vi "Run.vi"(8 "error in (no error)":errorcluster, 9 "Penalty":dbl, 10 "Map":i32[][](array[numeric]), 11 "Runner in":refnum<class "Rain.lvclass">) -> (0 "error out":errorcluster, 1 "Direction":T2, 2 "Action":T3, 3 "Runner out":refnum<class "Rain.lvclass">, 4 "Replicated":refnum<class "Square.lvclass">)   [LabVIEW 2015, in "Rain.lvclass"]
uses:
  Rain.lvclass
  Type Defs/Action Enum.ctl
  Type Defs/Direction Enum.ctl
  Square/Square.lvclass
  Carl/Formics/Attack Options.ctl
  SubVIs/Read-Only Globals.vi
  Carl/Common/Common.lvlib
  Type Defs/SB Type Defs.lvlib
  Carl/Formics/Formics.lvclass
panel:
  in  "Attack":T1
  # "NOTICE - YOU MUST NOT REMOVE THIS NOTICE. PER THE FOLLOWING LICENSE, YOU MAY REPRODUCE THIS SOFTWARE PROVIDED YOU FOLLOW THE TERMS\nOF THE LICENSE.\n\n---BEGIN BSD LICENSE (http://opensource.org/licenses/BSD-2-Clause)---\nCopyright (c) 2015, Endigit, Inc. <robert@endigit.com>\nAll rights reserved.\n\nRedistribution and use in source and binary forms, with or without modification, are permitted provided that the following conditions are met:\n\n1. Redistributions of source code must retain the above copyright notice, this list of conditions and the following disclaimer.\n\n2. Redistributions in binary form must reproduce the above copyright notice, this list of conditions and the following disclaimer in the documentation and/or other \nmaterials provided with the distribution.\n\nTHIS SOFTWARE IS PROVIDED BY THE COPYRIGHT HOLDERS AND CONTRIBUTORS \"AS IS\" AND ANY EXPRESS OR IMPLIED WARRANTIES, INCLUDING, BUT NOT \nLIMITED TO, THE IMPLIED WARRANTIES OF MERCHANTABILITY AND FITNESS FOR A PARTICULAR PURPOSE ARE DISCLAIMED. IN NO EVENT SHALL THE COPYRIGHT \nHOLDER OR CONTRIBUTORS BE LIABLE FOR ANY DIRECT, INDIRECT, INCIDENTAL, SPECIAL, EXEMPLARY, OR CONSEQUENTIAL DAMAGES (INCLUDING, BUT NOT \nLIMITED TO, PROCUREMENT OF SUBSTITUTE GOODS OR SERVICES; LOSS OF USE, DATA, OR PROFITS; OR BUSINESS INTERRUPTION) HOWEVER CAUSED AND ON \nANY THEORY OF LIABILITY, WHETHER IN CONTRACT, STRICT LIABILITY, OR TORT (INCLUDING NEGLIGENCE OR OTHERWISE) ARISING IN ANY WAY OUT OF THE USE \nOF THIS SOFTWARE, EVEN IF ADVISED OF THE POSSIBILITY OF SUCH DAMAGE.\n---END BSD LICENSE---"
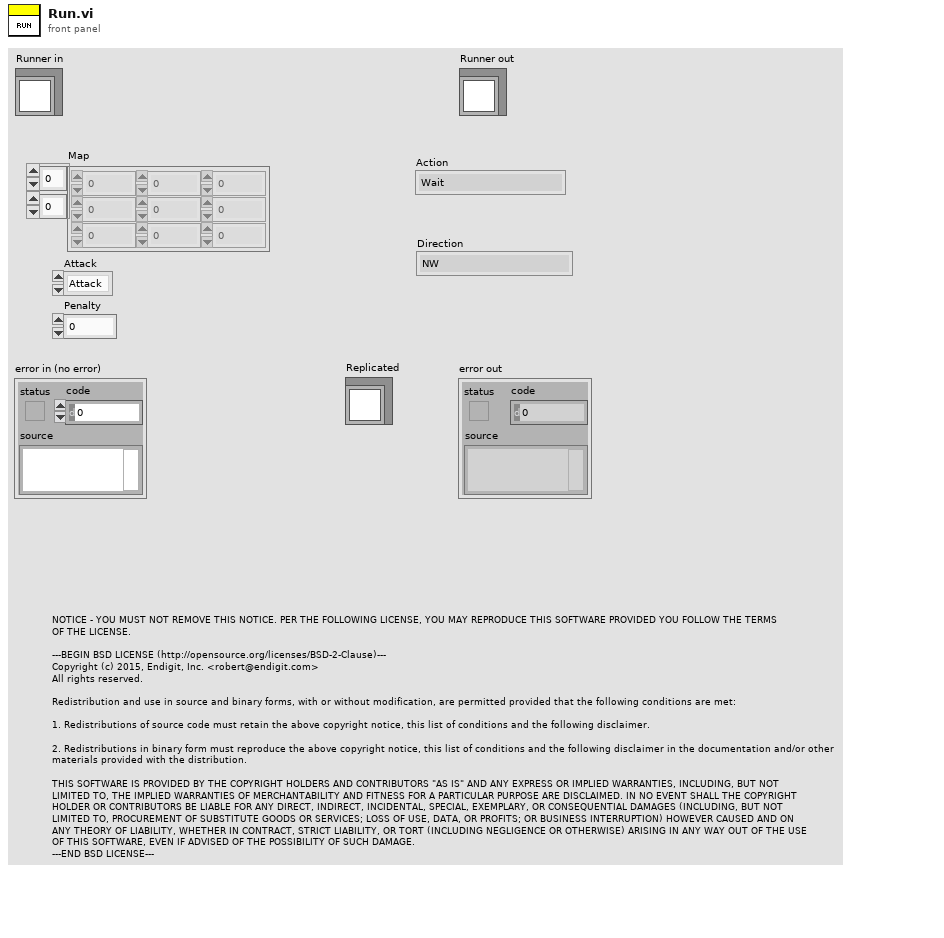
[diagram p1: front panel]
types:
  T1 = typedef "Formics.lvclass/Attack Options.ctl" = enum16{"Attack", "Run", "Distract"}
  T2 = typedef "SB Type Defs.lvlib/Direction Enum.ctl" = enum16{"NW", "N", "NE", "E", "SE", "S", "SW", "W"}
  T3 = typedef "SB Type Defs.lvlib/Action Enum.ctl" = enum16{"Wait", "Move", "Attack", "Replicate"}
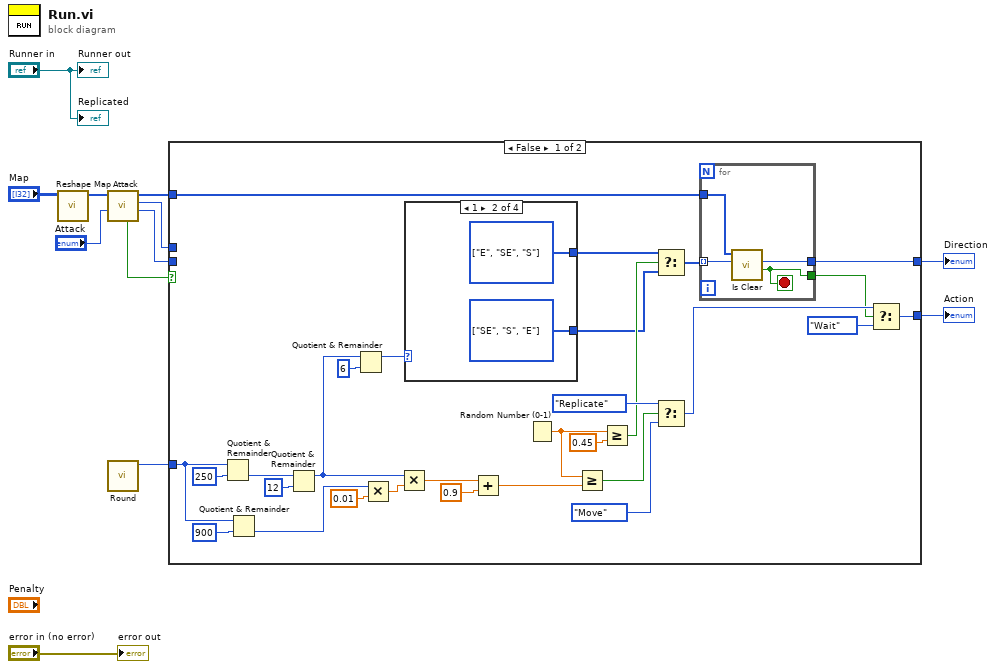
[diagram p0: block diagram]
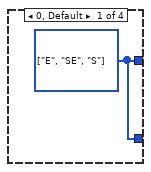
[diagram p2: hidden frame]
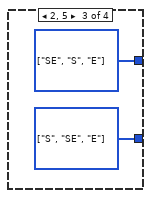
[diagram p3: hidden frame]
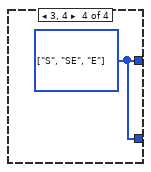
[diagram p4: hidden frame]
diagram:
  n1 = call "Reshape Map.vi"("Maze (0: Empty, -1: Enemy. >0: Teammate"="Map") -> ("Map"=w10:i32[])  [unwired: 9 in, 1 out]
  n2 = call "Attack.vi"("Attack?"="Attack", "Maze (0: Empty, -1: Enemy. >0: Teammate"=w10) -> ("Direction"=w8:i32, "Action"=w6:T3, "Maze (0: Empty, -1: Enemy. >0: Teammate 2"=w4:i32[], "Enemy Found?"=w9:bool)  [unwired: 4 in, 2 out]
  n3 = call "Round.vi"() -> ("Round"=w1:i32)  [unwired: 11 in]
  n4 = case shown="False" w9 {
    tunnel: w8 -> [_ w53]
    tunnel: [w34 w53] -> w7
    tunnel: w6 -> [_ w52]
    tunnel: [w38 w52] -> w5
    tunnel: w4 -> [w35 _]
    tunnel: w1 -> [w17 _]
    frame False {
      n5 = Quotient & Remainder(x=w17, y=250) -> (floor(x/y)=w25:i32)  [unwired: 1 out]
      n6 = Quotient & Remainder(x=w17, y=900) -> (floor(x/y)=w15:i32)  [unwired: 1 out]
      n7 = Quotient & Remainder(x=w25, y=12) -> (x-y*floor(x/y)=w19:i32)  [unwired: 1 out]
      n8 = Quotient & Remainder(x=w19, y=6) -> (x-y*floor(x/y)=w18:i32)  [unwired: 1 out]
      n9 = Multiply(x=w15, y=0.01) -> (x*y=w13:dbl)
      n10 = Multiply(x=w19, y=w13) -> (x*y=w24:dbl)
      n11 = case shown="1" w18 {
        tunnel: [w42 w44 w46 w47] -> w29
        tunnel: [w42 w43 w45 w47] -> w30
        frame 0, Default {
          w42 = T2[] [enum."E", enum."SE", enum."S"] items=["NW", "N", "NE", "E", "SE", "S", "SW", "W"]
        }
        frame 1 {
          w43 = T2[] [enum."SE", enum."S", enum."E"] items=["NW", "N", "NE", "E", "SE", "S", "SW", "W"]
          w44 = T2[] [enum."E", enum."SE", enum."S"] items=["NW", "N", "NE", "E", "SE", "S", "SW", "W"]
        }
        frame 2, 5 {
          w45 = T2[] [enum."S", enum."SE", enum."E"] items=["NW", "N", "NE", "E", "SE", "S", "SW", "W"]
          w46 = T2[] [enum."SE", enum."S", enum."E"] items=["NW", "N", "NE", "E", "SE", "S", "SW", "W"]
        }
        frame 3, 4 {
          w47 = T2[] [enum."S", enum."SE", enum."E"] items=["NW", "N", "NE", "E", "SE", "S", "SW", "W"]
        }
      }
      n12 = Add(x=w24, y=0.9) -> (x+y=w22:dbl)
      n13 = Random Number (0-1)() -> (number: 0 to 1=w27:dbl)
      n14 = Greater Or Equal?(x=w27, y=w22) -> (x >= y?=w33:bool)
      n15 = Greater Or Equal?(x=w27, y=0.45) -> (x >= y?=w31:bool)
      n16 = Select(t=w29, s=w31, f=w30) -> (s? t:f=w28:T2[])
      n17 = Select(t=Action_Enum."Replicate" ("Action"), s=w33, f=Action_Enum."Move" ("Action")) -> (s? t:f=w39:T3)
      n18 = for {
        tunnel: [w49] -> w37
        tunnel: w28 -> [w51] mode=indexing
        tunnel: w35 -> [w50]
        tunnel: [w48] -> w34
        stop <- w49 stop-if-true
        n19 = call "Is Clear.vi"("Direction"=w51, "Maze"=w50) -> ("Can Move?"=w49:bool, "Direction Out"=w48:T2)  [unwired: 7 in, 1 out]
      }
      n20 = Select(t=w39, s=w37, f=Action_Enum."Wait" ("Action")) -> (s? t:f=w38:T3)
    }
    frame True {
    }
  }
  "Action" <- w5
  "Direction" <- w7
  "error out" <- "error in (no error)"
  "Runner out" <- "Runner in"
  "Replicated" <- "Runner in"
